vi "Laser Feedback-PD ver.vi"() -> ()   [LabVIEW 2014]
uses:
  <vilib>/Analysis/NI_AALPro.lvlib
  <vilib>/Analysis/polynomials.llb/Scalar Polynomial Evaluation (DBL).vi
  <vilib>/addons/control/pid/NI_PID_pid.lvlib
  <vilib>/addons/control/pid/pid.llb/PID (DBL).vi
  Main-Stage-PI/(Global) Current handle and LaserPower_YCC.vi
  <vilib>/Analysis/NI_AALBase.lvlib
  <vilib>/Analysis/baseanly.llb/Mean (DBL).vi
  <vilib>/Utility/file.llb/Write To Spreadsheet File (DBL).vi
  <vilib>/DAQmx/read.llb/DAQmx Read (Analog 2D DBL NChan NSamp).vi
panel:
  in  "Save feedback data?":bool
  in  "PID gains 2":T1={"proportional gain (Kc)"=0.0171, "integral time (Ti, min)"=5e-06, "derivative time (Td, min)"=0.0014} {"derivative time (Td, min)" format="%#.6g"; "integral time (Ti, min)" format="%#.6g"; "proportional gain (Kc)" format="%#.6g"}
  in  "stop":bool
  out "Photodiode readout (mV)":dbl
  out "Set Laser power (mV)":dbl
  out "AOM (V)":dbl format="%.2f"
  out "Polynomial Coefficients":dbl[](array[numeric])
  in  "Tab Control":enum32{"Calibration curve", "Page 2"}(tab)
  out "XY Graph":T2(graph)
  out "Waveform Chart":dbl(graph)
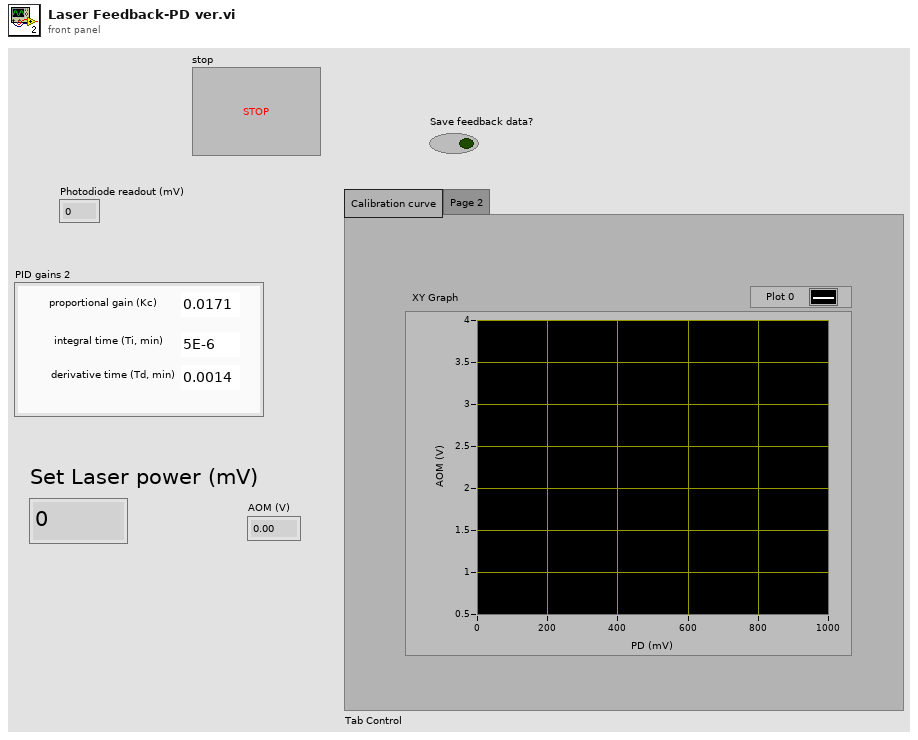
[diagram p1: front panel]
types:
  T1 = cluster{"proportional gain (Kc)":dbl, "integral time (Ti, min)":dbl, "derivative time (Td, min)":dbl}
  T2 = cluster{"Cal-PD (mV)":dbl[], "Best Polynomial Fit":dbl[]}[]
  T3 = cluster{"Cal-PD (mV)":dbl[], "Cal-AOM (V)":dbl[], "Best Polynomial Fit":dbl[], "Polynomial Coefficients":dbl[]}
  T4 = cluster{"Cal-PD (mV)":dbl[], "Cal-AOM (V)":dbl[]}
  T5 = cluster{"Cal-PD (mV)":dbl[], "Best Polynomial Fit":dbl[]}
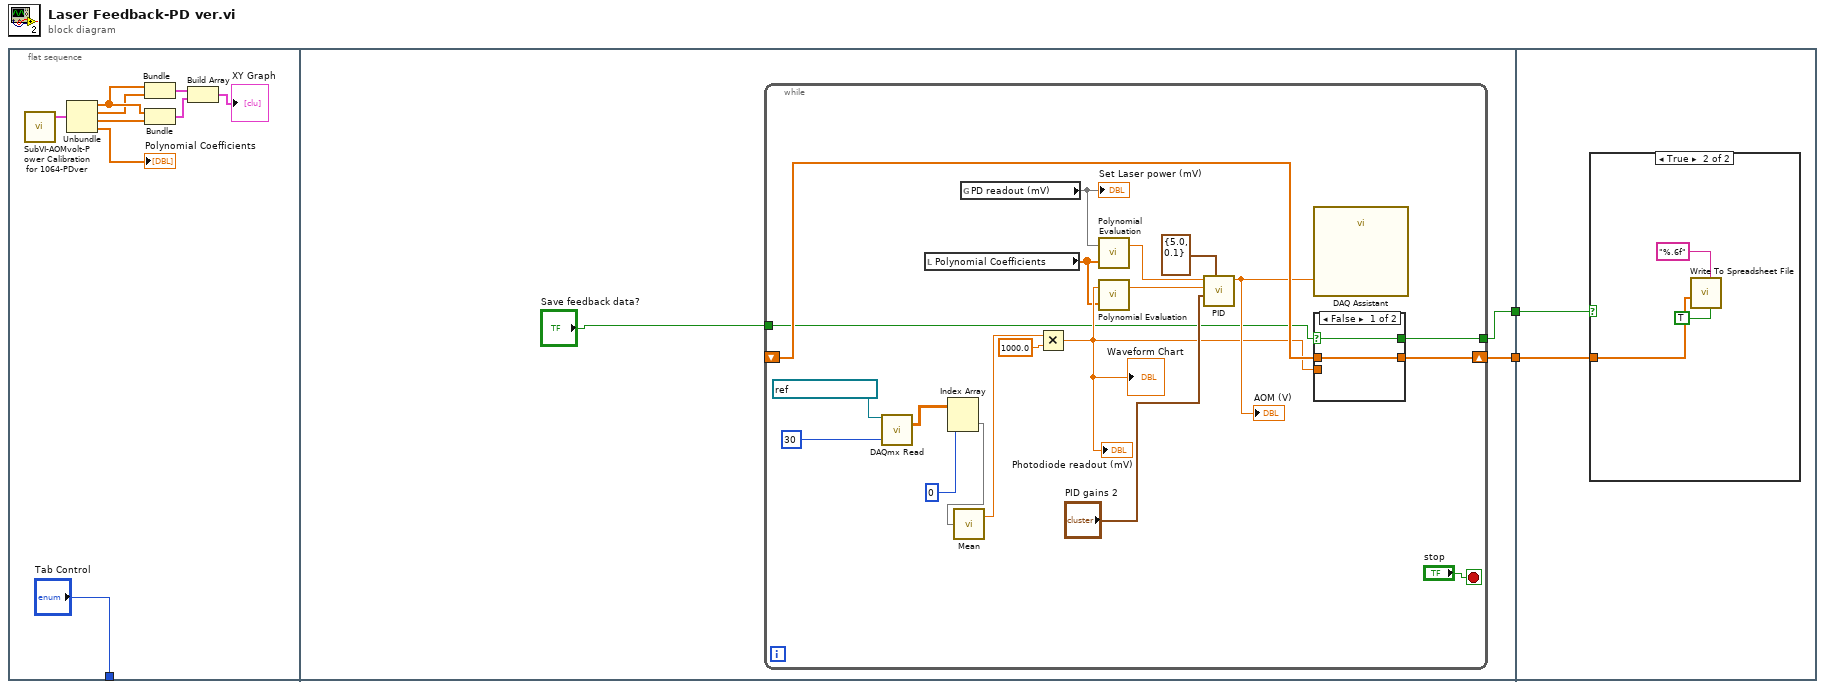
[diagram p0: block diagram]
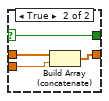
[diagram p2: hidden frame]
diagram:
  n1 = flat-sequence {
    tunnel: ["Tab Control"] -> _
    tunnel: [w13] -> w2
    tunnel: [w12] -> w1
    tunnel: w2 -> [w42]
    tunnel: w1 -> [w41]
    frame #0 {
      n2 = call "SubVI-AOMvolt-Power Calibration for 1064-PDver.vi"() -> ("output cluster"=w11:T3)  [unwired: 5 in, 1 out]
      n3 = Unbundle(w11) -> ("Cal-PD (mV)"=w10:dbl[], "Cal-AOM (V)"=w9:dbl[], "Best Polynomial Fit"=w8:dbl[], "Polynomial Coefficients"=→"Polynomial Coefficients":dbl[])
      n4 = Bundle("Cal-PD (mV)"=w10, "Cal-AOM (V)"=w9) -> (w6:T4)  [unwired: 1 in]
      n5 = Bundle("Cal-PD (mV)"=w10, "Best Polynomial Fit"=w8) -> (w5:T5)  [unwired: 1 in]
      n6 = Build Array(w6, w5) -> (→"XY Graph":T2)
    }
    frame #1 {
      n7 = while {
        tunnel: [w29] -> w13
        shift-right: [w28] -> w12
        shift-left: _ -> [w27]
        tunnel: "Save feedback data?" -> [w20]
        stop <- "stop" stop-if-true
        n8 = call-poly <vilib>:"DAQmx Read.vi"("task/channels in"=refnum<k21> "PD-read-Task", "number of samples per channel"=30) -> ("data"=w17:dbl[][])  [unwired: 11 in, 2 out]
        n9 = local read "Polynomial Coefficients"() -> (w21:dbl[])
        n10 = Index Array(array=w17, index (row)=0) -> (element=w15:dbl[])  [unwired: 1 in]
        n11 = call-poly <vilib>:"Mean.vi"("X"=w15) -> ("mean"=w22:dbl)  [unwired: 1 out]
        n12 = global read "(Global) Current handle and LaserPower_YCC.vi" "PD readout (mV)"() -> (w23)
        "Set Laser power (mV)" <- w23
        n13 = Multiply(x=w22, y=1000.0) -> (x*y=w24:dbl)
        "Photodiode readout (mV)" <- w24
        "Waveform Chart" <- w24
        n14 = call-poly <vilib>:"Polynomial Evaluation.vi"("P(x)"=w21, "a"=w23) -> ("P(a)"=w33:dbl)  [unwired: 1 out]
        n15 = call-poly <vilib>:"Polynomial Evaluation.vi"("P(x)"=w21, "a"=w24) -> ("P(a)"=w32:dbl)  [unwired: 1 out]
        n16 = call-poly <vilib>:"PID.vi"("output range"=cluster{"output high":dbl, "output low":dbl} {"output high"=5.0, "output low"=0.1}, "PID gains"="PID gains 2", "process variable"=w32, "setpoint"=w33) -> ("output"=w25:dbl)  [unwired: 6 in, 1 out]
        "AOM (V)" <- w25
        n17 = call "DAQ Assistant"("data"=w25) -> ()  [unwired: 17 in, 2 out]
        n18 = case shown="False" w20 {
          selector: w20 -> [w36 w40]
          tunnel: [w36 w40] -> w29
          tunnel: w24 -> [_ w38]
          tunnel: [w35 w37] -> w28
          tunnel: w27 -> [w35 w39]
          frame False {
          }
          frame True {
            n19 = Build Array (concatenate)(w39, w38) -> (w37:dbl[])
          }
        }
      }
    }
    frame #2 {
      n20 = case shown="True" w42 {
        tunnel: w41 -> [_ w45]
        frame False {
        }
        frame True {
          n21 = call-poly <vilib>:"Write To Spreadsheet File.vi"("transpose? (no:F)"=TRUE, "format (%.3f)"="%.6f", "1D data"=w45) -> ()  [unwired: 5 in, 1 out]
        }
      }
    }
  }
